vi "solar_cfg Write File (Str).vi"(0 "Config Path (*.ini)":path, 1 "Section (\"\" = Use Filename)":string, 2 "Comment":string, 5 "Key":string, 7 "Value in":string, 9 "Add Quotes? (T)":bool=TRUE, 11 "error in (no error)":errorcluster) -> (4 "Config Path out":path, 10 "Found?":bool, 15 "error out":errorcluster)   [LabVIEW 2018]
doc: "Write a value associated with a key to a specified section in the configuration file. Set a Comment (#...) to add a description after the key's value.\n\n[Section]\nKey = \"Value\" #Comment"
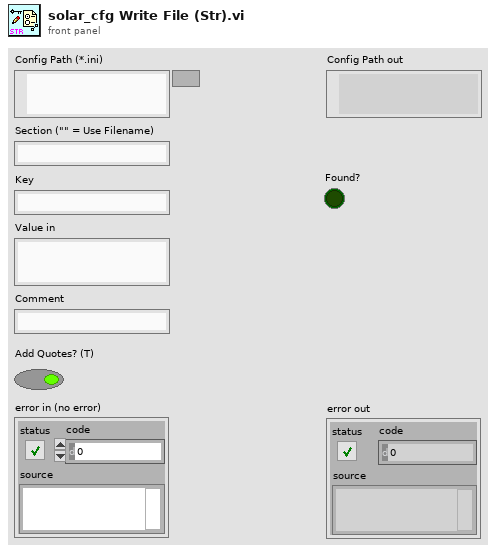
[diagram p1: front panel]
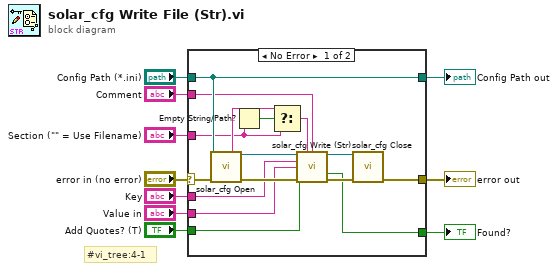
[diagram p0: block diagram]
diagram:
  # "#vi_tree:4-1"
  n1 = case shown="No Error" "error in (no error)" {
    selector: "error in (no error)" -> [w26 w28]
    tunnel: "Config Path (*.ini)" -> [w25 w27]
    tunnel: "Key" -> [w15 _]
    tunnel: [w20 w28] -> w7
    tunnel: "Section (\"\" = Use Filename)" -> [w11 _]
    tunnel: [w19 _] -> w5
    tunnel: [w25 w27] -> w4
    tunnel: "Value in" -> [w18 _]
    tunnel: "Comment" -> [w16 _]
    tunnel: "Add Quotes? (T)" -> [w17 _]
    frame No Error {
      n2 = call "solar_cfg Open.vi"("Config Path (*.ini)"=w25, "error in (no error)"=w26) -> ("Filename"=w13:string, "Config Refnum"=w23:refnum<data-value>, "error out"=w24:errorcluster)  [unwired: 10 in, 1 out]
      n3 = Empty String/Path?(string/path=w11) -> (empty?=w14:bool)
      n4 = Select(t=w13, s=w14, f=w11) -> (s? t:f=w12:string)
      n5 = call "solar_cfg Write (Str).vi"("Config Refnum"=w23, "Section"=w12, "Comment"=w16, "Key"=w15, "Value in"=w18, "Add Quotes? (T)"=w17, "error in (no error)"=w24) -> ("dup Config Refnum"=w21:refnum<data-value>, "Found?"=w19:bool, "error out"=w22:errorcluster)  [unwired: 6 in]
      n6 = call "solar_cfg Close.vi"("Config Refnum"=w21, "error in (no error)"=w22) -> ("error out"=w20:errorcluster)  [unwired: 12 in, 1 out]
    }
    frame Error {
    }
  }
  "error out" <- w7
  "Config Path out" <- w4
  "Found?" <- w5
